vi "ArduinoClose.vi"(1 "error in (no error)":errorcluster, 2 "VISA resource name":refnum<visa-resource-name>="COM24") -> (0 "error out":errorcluster)   [LabVIEW 2013, in "ArduinoControl.lvclass"]
uses:
  ArduinoControl.lvclass
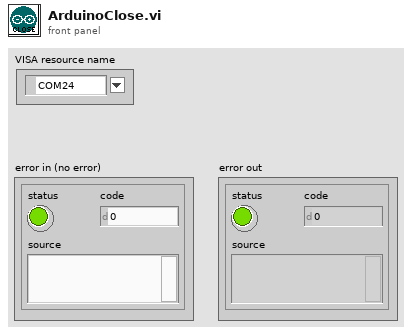
[diagram p1: front panel]
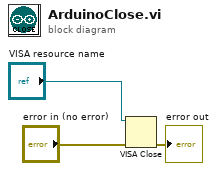
[diagram p0: block diagram]
diagram:
  n1 = VISA Close(VISA resource name="VISA resource name", error in (no error)="error in (no error)") -> (error out=→"error out":errorcluster)
